vi "Write guideStateTypes.vi"(8 "error in (no error)":errorcluster, 10 "guideStateTypes":T1, 11 "Guide in":refnum<class "Guide.lvclass">) -> (0 "error out":errorcluster, 3 "Guide out":refnum<class "Guide.lvclass">)   [LabVIEW 2014, in "TCSDataDefinitions.lvlib" / "TCSCommand.lvlib" / "GuiderCommands.lvlib" / "Guide.lvclass"]
uses:
  Guide.lvclass
  Enumerations/GuideStateTypes.ctl
  Guide.lvclass/Guide.ctl
  TCSCommand.lvlib
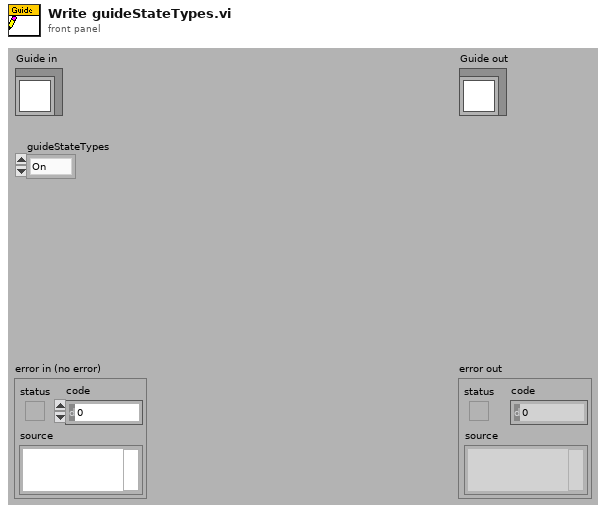
[diagram p1: front panel]
types:
  T1 = typedef "TCSDataDefinitions.lvlib/TCSCommand.lvlib/GuideStateTypes.ctl" = enum16{"On", "Off"}
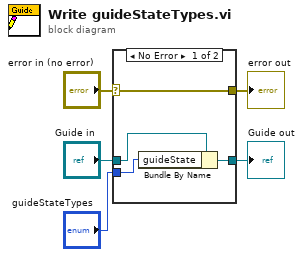
[diagram p0: block diagram]
diagram:
  n1 = case shown="No Error" "error in (no error)" {
    selector: "error in (no error)" -> [w9 w10]
    tunnel: [w9 w10] -> w4
    tunnel: [w7 w11] -> w2
    tunnel: "Guide in" -> [w8 w11]
    tunnel: "guideStateTypes" -> [w6 _]
    frame No Error {
      n2 = Bundle By Name(cluster=w8, "guideState"=w6) -> (w7:refnum<class "Guide.lvclass">)
    }
    frame Error {
    }
  }
  "error out" <- w4
  "Guide out" <- w2
